vi "Get Result.vi"(8 "error in (no error)":errorcluster, 11 "AverageCollector1D in":refnum<class "AverageCollector1D.lvclass">) -> (0 "error out":errorcluster, 2 "Collected Result out":refnum<class "AbstractData.lvclass">, 3 "AverageCollector1D out":refnum<class "AverageCollector1D.lvclass">)   [LabVIEW 2014, in "AverageCollector1D.lvclass"]
uses:
  AverageCollector1D.lvclass
  Framework/Model/Data/AbstractData/AbstractData.lvclass
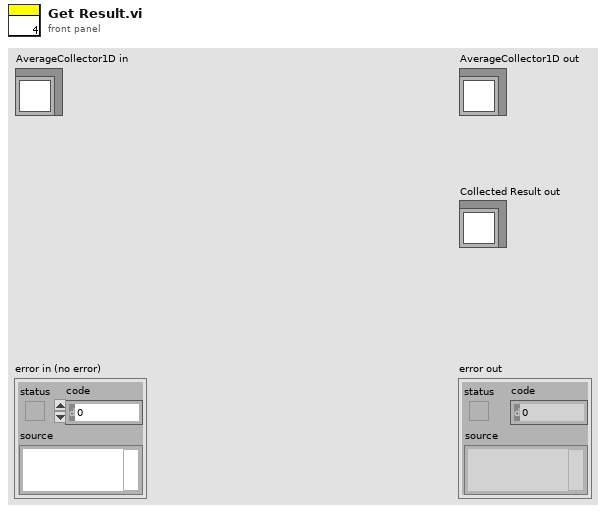
[diagram p1: front panel]
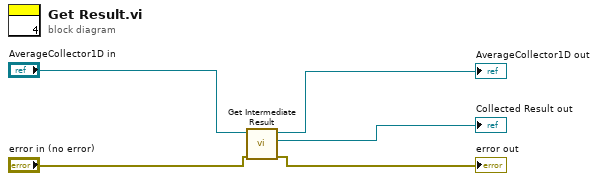
[diagram p0: block diagram]
diagram:
  n1 = call-dynamic "Get Intermediate Result.vi"("error in (no error)"="error in (no error)", "AverageCollector1D in"="AverageCollector1D in") -> ("error out"=→"error out":errorcluster, "AbstractData.lvclass"=→"Collected Result out":refnum<class "AbstractData.lvclass">, "AverageCollector1D out"=→"AverageCollector1D out":refnum<class "AverageCollector1D.lvclass">)  [unwired: 7 in]
